vi "SwerveAngleEncoderConversion.vi"(11 "Voltage":dbl) -> (3 "Angle":dbl)   [LabVIEW 2017]
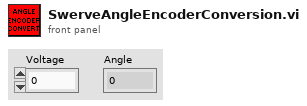
[diagram p1: front panel]
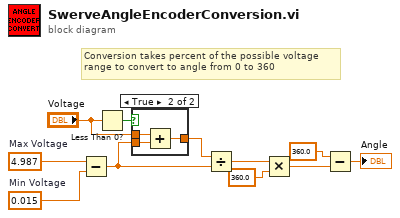
[diagram p0: block diagram]
diagram:
  w3 = 0.015  # Min Voltage
  w4 = 4.987  # Max Voltage
  # "Conversion takes percent of the possible voltage\nrange to convert to angle from 0 to 360"
  n1 = Subtract(x=w4, y=w3) -> (x-y=w1:dbl)
  n2 = Less Than 0?(x="Voltage") -> (x < 0?=w7:bool)
  n3 = case shown="True" w7 {
    tunnel: "Voltage" -> [w12 w15]
    tunnel: w1 -> [_ w13]
    tunnel: [w12 w14] -> w2
    frame False {
    }
    frame True {
      n4 = Add(x=w15, y=w13) -> (x+y=w14:dbl)
    }
  }
  n5 = Divide(x=w2, y=w1) -> (x/y=w9:dbl)
  n6 = Multiply(x=w9, y=360.0) -> (x*y=w5:dbl)
  n7 = Subtract(x=360.0, y=w5) -> (x-y=→"Angle":dbl)
